vi "For.vi"() -> ()   [LabVIEW 2020]
panel:
  out "Number (0 to 1)":dbl
  out "Numeric 2":i32
  in  "Control de iteracion":i32
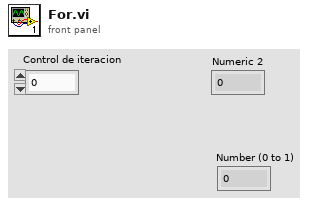
[diagram p1: front panel]
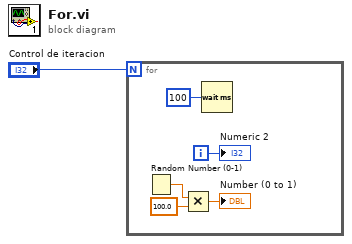
[diagram p0: block diagram]
diagram:
  n1 = for {
    N: "Control de iteracion" -> [_]
    i -> [w6]
    n2 = Random Number (0-1)() -> (number: 0 to 1=w3:dbl)
    n3 = Multiply(x=w3, y=100.0) -> (x*y=→"Number (0 to 1)":dbl)
    n4 = Wait (ms)(milliseconds to wait=100) -> ()  [unwired: 1 out]
    "Numeric 2" <- w6
  }
